vi "Mouse Down.vi"(8 "error in (no error)":errorcluster, 10 "Delay in ms (10)":u32=10, 11 "Button":i32) -> (0 "error out":errorcluster)   [LabVIEW 2020, in "MacroAssert.lvlib"]
uses:
  MacroAssert.lvlib
  user32.dll
  fdaed37b-1ab6-437a-8e89-3a5b05fa2717.vi
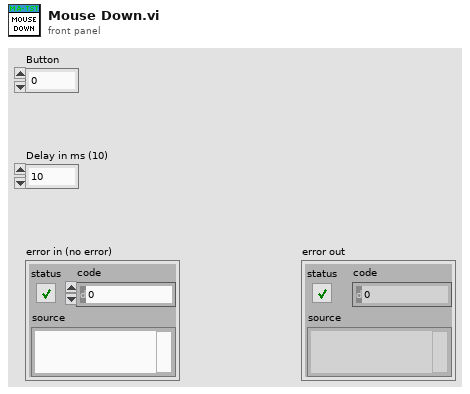
[diagram p1: front panel]
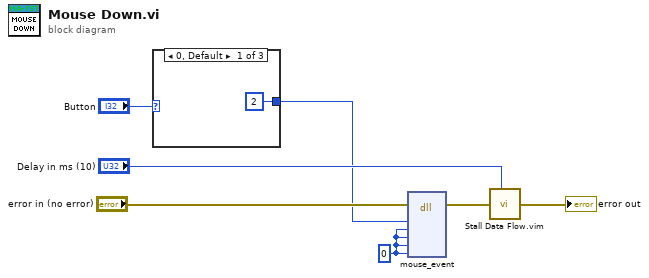
[diagram p0: block diagram]
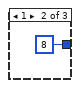
[diagram p2: hidden frame]
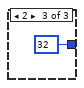
[diagram p3: hidden frame]
diagram:
  w7 = 0 ("dx")
  n1 = case shown="0, Default" "Button" {
    tunnel: [2 8 32] -> w1
    frame 0, Default {
    }
    frame 1 {
    }
    frame 2 {
    }
  }
  n2 = dll-call lib="user32.dll" fn="mouse_event"(error in="error in (no error)", "flags"=w1, "dx"=w7, "dx"=w7, "data"=w7, "ptr"=w7) -> (error out=w4:errorcluster)  [unwired: 8 in, 1 out]
  n3 = call "Stall Data Flow.vim"("value in"=w4, "milliseconds to wait"="Delay in ms (10)") -> ("value out"=→"error out":errorcluster)  [unwired: 1 out]
